vi "Publish.vi"(8 "error in (no error)":errorcluster, 9 "Message to be published":string=" Message", 11 "connection ID":refnum<k5>) -> (0 "error out":errorcluster, 3 "connection ID out":refnum<k5>)   [LabVIEW 2013, in "IOTFoundation.lvlib"]
uses:
  IOTFoundation.lvlib
  Controls/MessageType.ctl
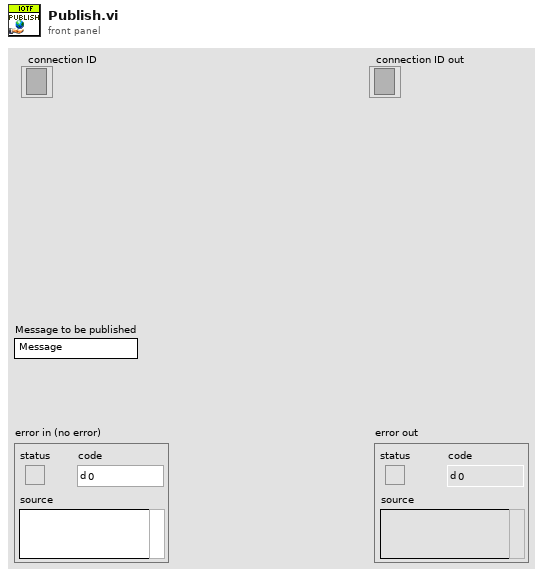
[diagram p1: front panel]
types:
  T1 = typedef "IOTFoundation.lvlib/MessageType.ctl" = enum32{"Reserved", "CONNECT", "CONNACK", "PUBLISH", "PUBACK", "PUBREC", "PUBREL", "PUBCOMP", "SUBSCRIBE", "SUBACK", "UNSUBSCRIBE", "UNSUBACK", "PINGREQ", "PINGRESP", "DISCONNECT", "Reserved2"}
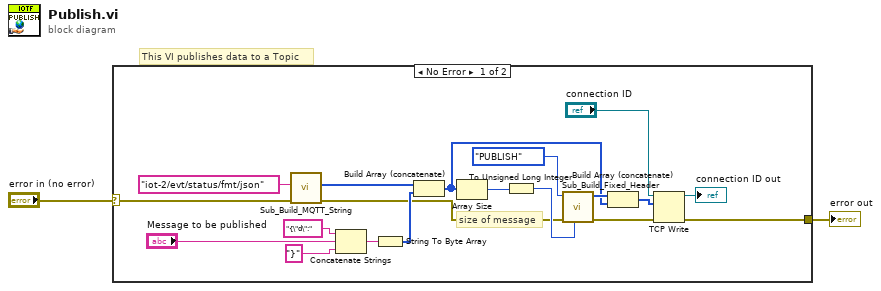
[diagram p0: block diagram]
diagram:
  # "This VI publishes data to a Topic"
  n1 = case shown="No Error" "error in (no error)" {
    selector: "error in (no error)" -> [w13 w22]
    tunnel: [w9 w22] -> w1
    frame No Error {
      # "size of message"
      n2 = call "Sub_Build_MQTT_String.vi"("error in (no error)"=w13, "String to be encoded"="iot-2/evt/status/fmt/json") -> ("error out"=w3:errorcluster, "UTF8 Byte Array"=w12:u8[])  [unwired: 8 in]
      n3 = Concatenate Strings("{\"d\":", "Message to be published", "}") -> (w5:string)
      n4 = String To Byte Array(string=w5) -> (unsigned byte array=w4:u8[])
      n5 = Build Array (concatenate)(w12, w4) -> (w17:u8[])
      n6 = Array Size(array=w17) -> (size(s)=w19:i32)
      n7 = To Unsigned Long Integer(number=w19) -> (unsigned 32bit integer=w20:u32)
      n8 = call "Sub_Build_Fixed_Header.vi"("Remaining Length"=w20, "error in (no error)"=w3, "MessageType"=MessageType."PUBLISH") -> ("error out"=w10:errorcluster, "Fixed Header"=w18:u8[])  [unwired: 7 in]
      n9 = Build Array (concatenate)(w18, w17) -> (w8:u8[])
      n10 = TCP Write(connection ID="connection ID", data in=w8, error in (no error)=w10) -> (connection ID out=→"connection ID out":refnum<k5>, error out=w9:errorcluster)  [unwired: 1 in, 1 out]
    }
    frame Error {
    }
  }
  "error out" <- w1
